vi "OICB-Set LED's.vi"(8 "error in (no error)":errorcluster, 11 "LED Outputs":T1) -> (0 "error out":errorcluster)   [LabVIEW 2015]
uses:
  LED_Output_TypeDef.ctl
  <vilib>/Rock Robotics/Network Tables/NT Write String.vi
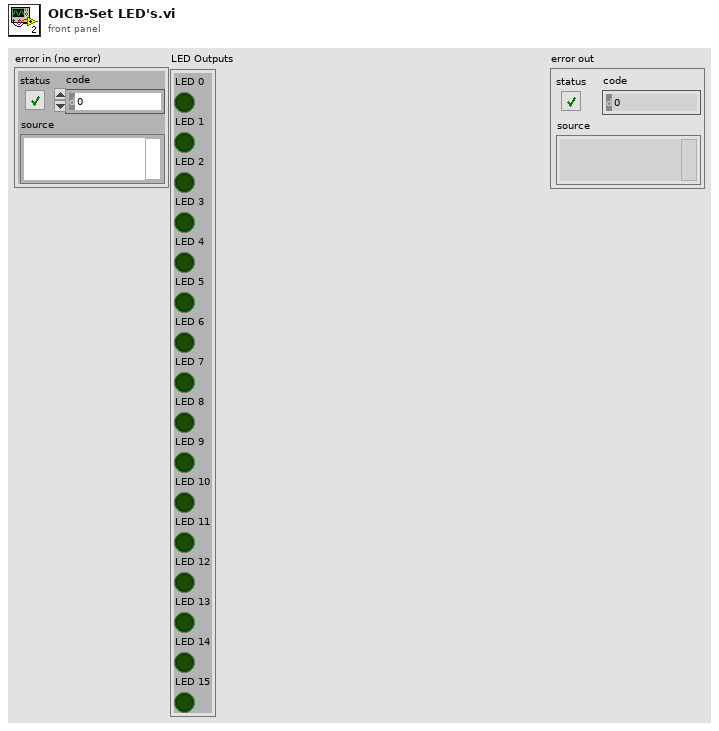
[diagram p1: front panel]
types:
  T1 = typedef "LED_Output_TypeDef.ctl" = cluster{"LED 0":bool, "LED 1":bool, "LED 2":bool, "LED 3":bool, "LED 4":bool, "LED 5":bool, "LED 6":bool, "LED 7":bool, "LED 8":bool, "LED 9":bool, "LED 10":bool, "LED 11":bool, "LED 12":bool, "LED 13":bool, "LED 14":bool, "LED 15":bool}
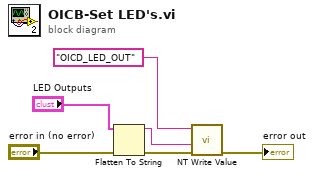
[diagram p0: block diagram]
diagram:
  n1 = Flatten To String(anything="LED Outputs", error in (no error)="error in (no error)") -> (data string=w5:string, error out=w4:errorcluster)  [unwired: 2 in, 1 out]
  n2 = call-poly <vilib>:"NT Write Value.vi"("error in"=w4, "String"=w5, "Name"="OICD_LED_OUT") -> ("error out"=→"error out":errorcluster)  [unwired: 8 in]
